vi "Write Specifications.vi"(10 "Specifications":string="C:\\Sandbox\\Supporting Materials\\Specifications\\specsheet.specs", 11 "niDigital in":refnum<class "niDigital.lvclass">) -> (3 "niDigital out":refnum<class "niDigital.lvclass">)   [LabVIEW 2020, in "niDigital.lvclass"]
uses:
  niDigital.lvclass
  niDigital.lvclass/niDigital.ctl
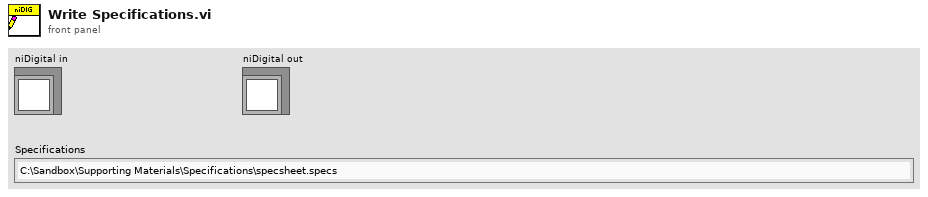
[diagram p1: front panel]
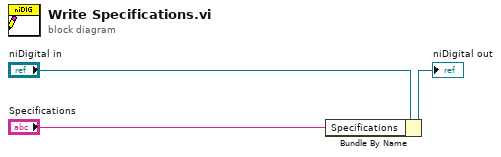
[diagram p0: block diagram]
diagram:
  n1 = Bundle By Name(cluster="niDigital in", "Specifications"="Specifications") -> (→"niDigital out":refnum<class "niDigital.lvclass">)
